vi "multiplexer.vi"() -> ()   [LabVIEW 2014]
uses:
  <vilib>/GPower/Numeric/GPNumeric.lvlib
panel:
  in  "LogFile":path
  in  "Logging Enabled?":bool
  # "\"mplexer data in\" - queue to receive data from sensors\n\"mplexer msg in\" - queue to send messages to multiplexer\n\"mplexer clock\" - notifier that will sound off every 25 ms, with an incrementing counter as a value; use it if you like.  Also, it will be canceled 10 ms after it sounds.\n\n\n\"mplexer msg out\" - none of your business!  (holds our subscribers - internal queue)"
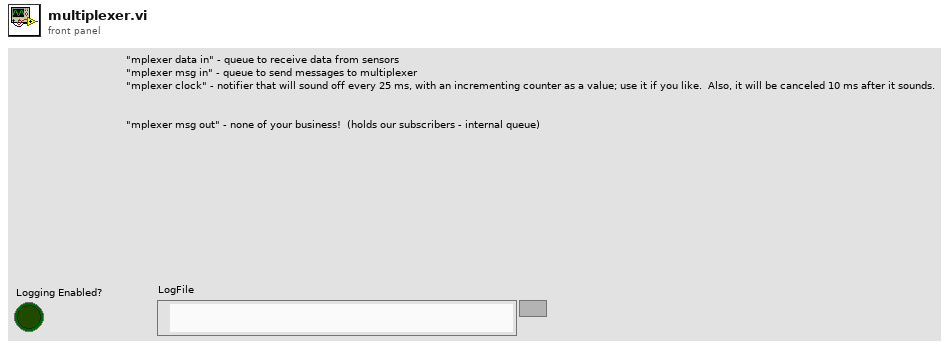
[diagram p1: front panel]
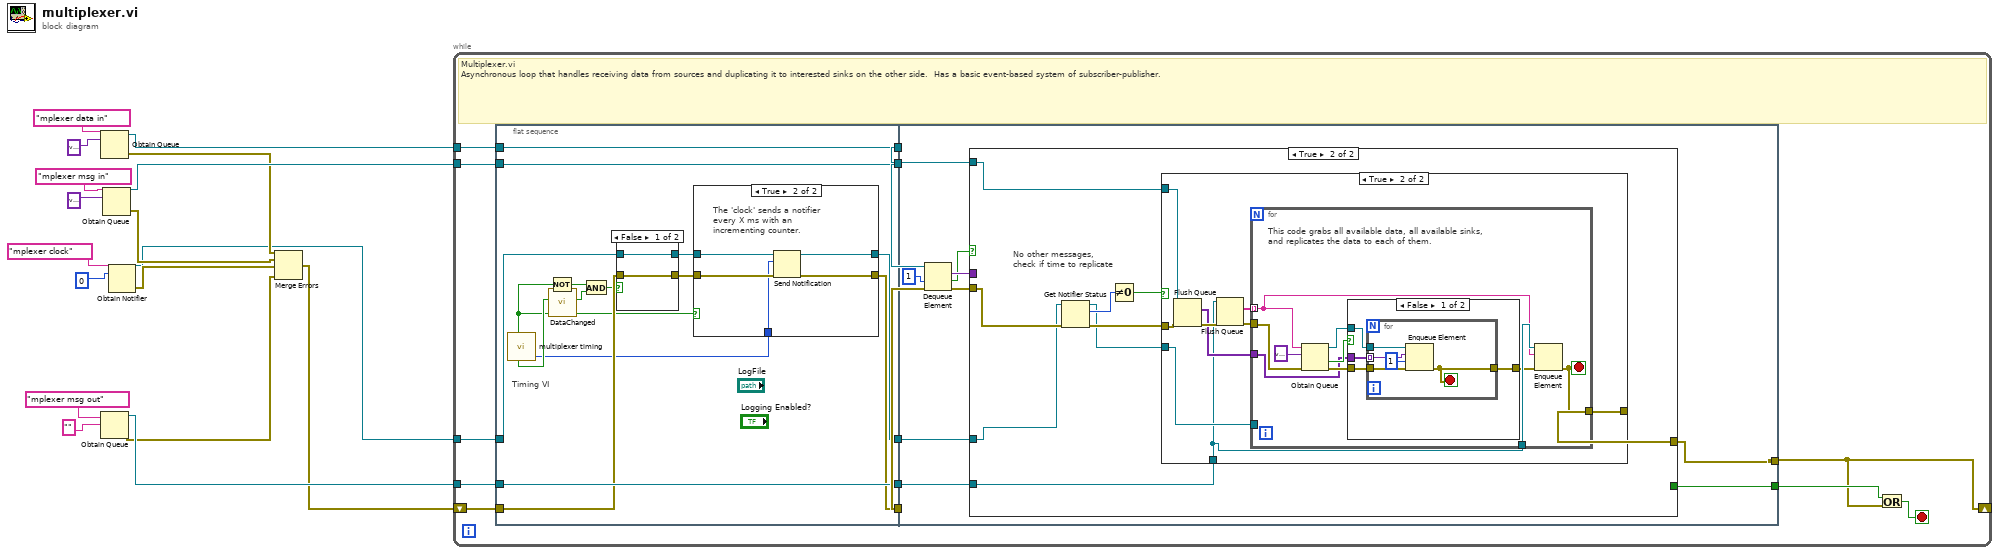
[diagram p0: block diagram]
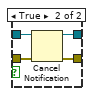
[diagram p2: hidden frame]
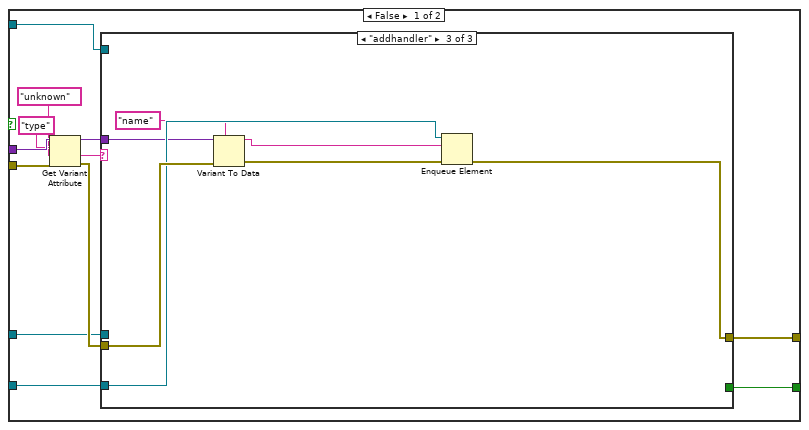
[diagram p4: hidden frame]
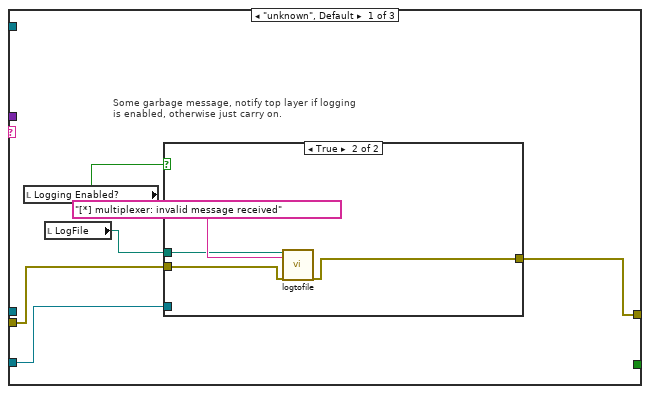
[diagram p5: hidden frame]
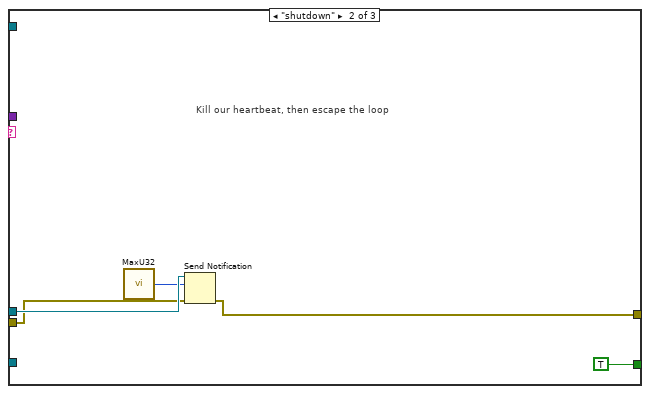
[diagram p7: hidden frame]
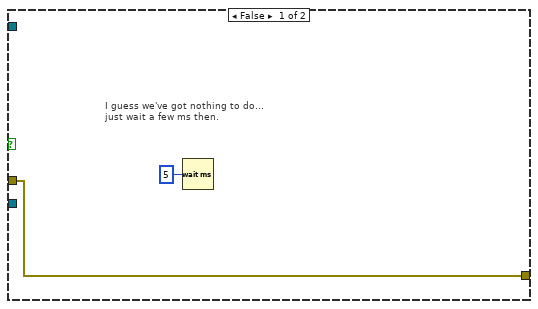
[diagram p8: hidden frame]
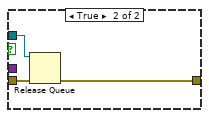
[diagram p9: hidden frame]
diagram:
  n1 = Obtain Queue(name (unnamed)="mplexer data in", element data type=variant) -> (queue out=w16:refnum<queue>, error out=w7:errorcluster)  [unwired: 3 in, 1 out]
  n2 = Obtain Queue(name (unnamed)="mplexer msg out", element data type="") -> (queue out=w13:refnum<queue>, error out=w1:errorcluster)  [unwired: 3 in, 1 out]
  n3 = Obtain Queue(name (unnamed)="mplexer msg in", element data type=variant) -> (queue out=w14:refnum<queue>, error out=w6:errorcluster)  [unwired: 3 in, 1 out]
  n4 = Obtain Notifier(name (unnamed)="mplexer clock", notification data type=u32 0) -> (notifier out=w3:refnum<notifier>, error out=w5:errorcluster)  [unwired: 2 in, 1 out]
  n5 = Merge Errors(w7, w6, w5, w1) -> (w4:errorcluster)
  n6 = while {
    tunnel: w16 -> [w20]
    shift-right: [w18] -> _
    shift-left: w4 -> [w28]
    tunnel: w14 -> [w25]
    tunnel: w13 -> [w26]
    tunnel: w3 -> [w23]
    stop <- w30 stop-if-true
    # "Multiplexer.vi\nAsynchronous loop that handles receiving data from sources and duplicating it to interested sinks on the other side.  Has a basic event-based system of subscriber-publisher."
    n7 = flat-sequence {
      tunnel: w28 -> [w40]
      tunnel: [w43] -> w29
      tunnel: [w44] -> w27
      tunnel: w26 -> [w44]
      tunnel: w25 -> [w45]
      tunnel: [w45] -> w24
      tunnel: w23 -> [w41]
      tunnel: [w32] -> w22
      tunnel: [w42] -> w21
      tunnel: w20 -> [w42]
      tunnel: w29 -> [w68]
      tunnel: w27 -> [w66]
      tunnel: w24 -> [w64]
      tunnel: [w62] -> w18
      tunnel: w22 -> [w61]
      tunnel: w21 -> [w60]
      tunnel: [w59] -> w19
      frame #0 {
        # "Timing VI"
        n8 = call "multiplexer timing.vi"() -> ("Clock Tick"=w36:bool, "Latch"=w37:bool, "Clock Counter"=w31:u32)  [unwired: 4 in, 2 out]
        n9 = Not(x=w36) -> (.not. x?=w35:bool)
        n10 = call <vilib>:"DataChanged.vi"("Data"=w37) -> ("Data changed?"=w34:bool)  [unwired: 10 in]
        n11 = And(x=w35, y=w34) -> (x .and. y?=w33:bool)
        n12 = case shown="False" w33 {
          tunnel: w41 -> [w46 w51]
          tunnel: w40 -> [w47 w50]
          tunnel: [w47 w49] -> w38
          tunnel: [w46 w48] -> w39
          frame False {
          }
          frame True {
            n13 = Cancel Notification(0:w51, 3:w50) -> (8:w48:refnum<notifier>, 11:w49:errorcluster)  [unwired: 1 out]
          }
        }
        n14 = case shown="True" w36 {
          tunnel: w39 -> [w53 w58]
          tunnel: [w52 w57] -> w43
          tunnel: w38 -> [w52 w56]
          tunnel: [w53 w55] -> w32
          tunnel: w31 -> [_ w54]
          frame False {
          }
          frame True {
            # "The 'clock' sends a notifier\nevery X ms with an\nincrementing counter."
            n15 = Send Notification(notification=w54, notifier=w58, error in (no error)=w56) -> (notifier out=w55:refnum<notifier>, error out=w57:errorcluster)
          }
        }
      }
      frame #1 {
        n16 = Dequeue Element(queue=w64, timeout in ms (-1)=1) -> (element=w65:variant, timed out?=w63:bool)  [unwired: 1 in, 2 out]
        n17 = case shown="True" w63 {
          tunnel: w68 -> [w78 w108]
          tunnel: w65 -> [w80 _]
          tunnel: w66 -> [w74 w104]
          tunnel: [w73 w103] -> w62
          tunnel: w61 -> [w71 w107]
          tunnel: w60 -> [w70 w106]
          tunnel: [w69 _] -> w59
          frame False {
            n18 = Get Variant Attribute(Variant=w80, name="type", default value (empty Variant)="unknown", error in=w78) -> (duplicate Variant=w72:variant, value=w75:string, error out=w76:errorcluster)  [unwired: 1 out]
            n19 = case shown="\"addhandler\"" w75 {
              tunnel: w76 -> [w84 w94 w102]
              tunnel: w74 -> [w85 _ w101]
              tunnel: [w83 w92 w100] -> w73
              tunnel: w72 -> [_ _ w98]
              tunnel: w71 -> [_ w95 _]
              tunnel: w70 -> [_ _ _]
              tunnel: [_ TRUE _] -> w69
              frame "unknown", Default {
                # "Some garbage message, notify top layer if logging \nis enabled, otherwise just carry on."
                n20 = local read "Logging Enabled?"() -> (w82:bool)
                n21 = local read "LogFile"() -> (w81:path)
                n22 = case shown="True" w82 {
                  tunnel: w85 -> [_ _]
                  tunnel: w84 -> [w86 w88]
                  tunnel: [w86 w87] -> w83
                  tunnel: w81 -> [_ w89]
                  frame False {
                  }
                  frame True {
                    n23 = call "logtofile.vi"("LogFile"=w89, "text"="[*] multiplexer: invalid message received", "error in (no error)"=w88) -> ("error out"=w87:errorcluster)  [unwired: 16 in]
                  }
                }
              }
              frame "shutdown" {
                # "Kill our heartbeat, then escape the loop"
                n24 = call <vilib>:"MaxU32.vi"() -> ("Maximum value"=w93:u32)
                n25 = Send Notification(notification=w93, notifier=w95, error in (no error)=w94) -> (error out=w92:errorcluster)  [unwired: 1 out]
              }
              frame "addhandler" {
                n26 = Variant To Data(error in=w102, type="name" ("name"), Variant=w98) -> (data=w97:string, error out=w96:errorcluster)
                n27 = Enqueue Element(queue=w101, element=w97, error in (no error)=w96) -> (error out=w100:errorcluster)  [unwired: 1 in, 2 out]
              }
            }
          }
          frame True {
            # "No other messages,\ncheck if time to replicate"
            n28 = Get Notifier Status(notifier=w107, error in (no error)=w108) -> (notifier out=w105:refnum<notifier>, current notification=w111:u32, error out=w109:errorcluster)  [unwired: 2 out]
            n29 = Not Equal To 0?(x=w111) -> (x != 0?=w110:bool)
            n30 = case shown="True" w110 {
              tunnel: w109 -> [w113 w119]
              tunnel: w106 -> [_ w120]
              tunnel: [w113 w116] -> w103
              tunnel: w105 -> [_ w115]
              tunnel: w104 -> [_ w114]
              frame False {
                # "I guess we've got nothing to do...\njust wait a few ms then."
                n31 = Wait (ms)(milliseconds to wait=u32 5) -> ()  [unwired: 1 out]
              }
              frame True {
                n32 = Flush Queue(queue=w120, error in (no error)=w119) -> (remaining elements=w117:variant[], error out=w118:errorcluster)  [unwired: 1 out]
                n33 = Flush Queue(queue=w114, error in (no error)=w118) -> (remaining elements=w121:string[], error out=w122:errorcluster)  [unwired: 1 out]
                n34 = for {
                  tunnel: w122 -> [w132]
                  tunnel: w121 -> [w125] mode=indexing
                  tunnel: w115 -> [_]
                  tunnel: w117 -> [w127]
                  tunnel: [w123] -> w116
                  tunnel: w114 -> [w126]
                  stop <- w123 stop-if-true
                  # "This code grabs all available data, all available sinks,\nand replicates the data to each of them."
                  n35 = Obtain Queue(name (unnamed)=w125, element data type=variant, error in (no error)=w132) -> (queue out=w128:refnum<queue>, created new?=w130:bool, error out=w129:errorcluster)  [unwired: 2 in]
                  n36 = case shown="False" w130 {
                    tunnel: w129 -> [w134 w143]
                    tunnel: w128 -> [w135 w144]
                    tunnel: [w133 w142] -> w124
                    tunnel: w127 -> [w136 _]
                    frame False {
                      n37 = for {
                        tunnel: w136 -> [w141] mode=indexing
                        tunnel: w135 -> [w140]
                        tunnel: w134 -> [w139]
                        tunnel: [w138] -> w133
                        stop <- w138 stop-if-true
                        n38 = Enqueue Element(queue=w140, element=w141, timeout in ms (-1)=1, error in (no error)=w139) -> (error out=w138:errorcluster)  [unwired: 2 out]
                      }
                    }
                    frame True {
                      n39 = Release Queue(queue=w144, error in (no error)=w143) -> (error out=w142:errorcluster)  [unwired: 1 in, 2 out]
                    }
                  }
                  n40 = Enqueue Element(queue=w126, element=w125, error in (no error)=w124) -> (error out=w123:errorcluster)  [unwired: 1 in, 2 out]
                }
              }
            }
          }
        }
      }
    }
    n41 = Or(x=w19, y=w18) -> (x .or. y?=w30:bool)
  }
